vi "Array to VCluster.vi"(8 "错误输入":errorcluster, 10 "Array":variant) -> (0 "错误输出":errorcluster, 2 "VCluster":variant)   [LabVIEW 2012, in "TD Tools.lvlib"]
uses:
  TD Tools.lvlib
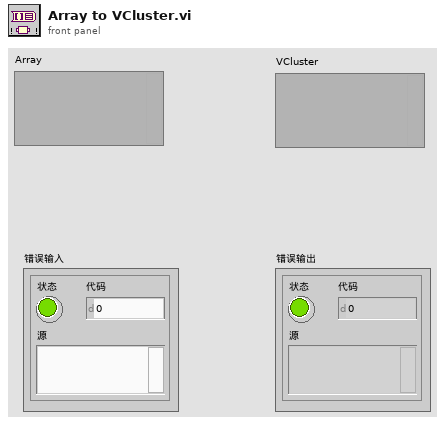
[diagram p1: front panel]
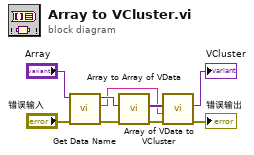
[diagram p0: block diagram]
diagram:
  n1 = call "Get Data Name.vi"("错误输入"="错误输入", "Data"="Array") -> ("错误输出"=w7:errorcluster, "Data Name"=w4:string, "Data dup"=w6:variant)  [unwired: 7 in]
  n2 = call "Array to Array of VData.vi"("错误输入"=w7, "MultiD Array"=w6) -> ("错误输出"=w3:errorcluster, "1D Array of Variants"=w5:variant[])  [unwired: 8 in]
  n3 = call "Array of VData to VCluster.vi"("error in (no error)"=w3, "Cluster Name"=w4, "Array"=w5) -> ("error out"=→"错误输出":errorcluster, "VCluster"=→"VCluster":variant)  [unwired: 7 in]
